vi "Add Colors.vi"(9 "Factor (1)":dbl=1.0, 10 "Color in":u32(colorbox), 11 "color":u32(colorbox)) -> (3 "Color out":u32(colorbox))   [LabVIEW 2025]
doc: "Adds two colors together and applies a factor (brightness) to the result."
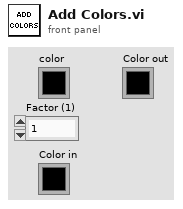
[diagram p1: front panel]
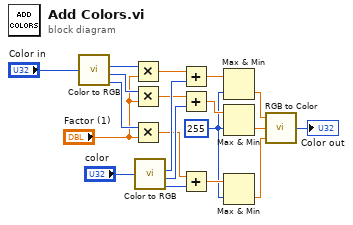
[diagram p0: block diagram]
diagram:
  w18 = u8 255 ("y")
  n1 = call <vilib>:"Color to RGB.vi"("Color"="Color in") -> ("R"=w8:u8, "G"=w9:u8, "B"=w10:u8)  [unwired: 1 out]
  n2 = Multiply(x=w8, y="Factor (1)") -> (x*y=w4:dbl)
  n3 = Multiply(x=w9, y="Factor (1)") -> (x*y=w3:dbl)
  n4 = Multiply(x=w10, y="Factor (1)") -> (x*y=w2:dbl)
  n5 = call <vilib>:"Color to RGB.vi"("Color"="color") -> ("R"=w12:u8, "G"=w13:u8, "B"=w14:u8)  [unwired: 1 out]
  n6 = Add(x=w4, y=w12) -> (x+y=w11:dbl)
  n7 = Add(x=w3, y=w13) -> (x+y=w19:dbl)
  n8 = Add(x=w2, y=w14) -> (x+y=w20:dbl)
  n9 = Max & Min(x=w11, y=w18) -> (min(x,y)=w7:dbl)  [unwired: 1 out]
  n10 = Max & Min(x=w19, y=w18) -> (min(x,y)=w6:dbl)  [unwired: 1 out]
  n11 = Max & Min(x=w20, y=w18) -> (min(x,y)=w5:dbl)  [unwired: 1 out]
  n12 = call <vilib>:"RGB to Color.vi"("B"=w5, "G"=w6, "R"=w7) -> ("Color"=→"Color out":u32)
